vi "Write Card #.vi"(8 "error in (no error)":errorcluster, 10 "Card #":dbl, 11 "Universal Card in":refnum<class "Universal Card.lvclass">) -> (0 "error out":errorcluster, 3 "Universal Card out":refnum<class "Universal Card.lvclass">)   [LabVIEW 2012, in "Universal Power Meter.lvlib" / "Universal Card.lvclass"]
uses:
  Universal Card.lvclass
  Universal Card.lvclass/Universal Card.ctl
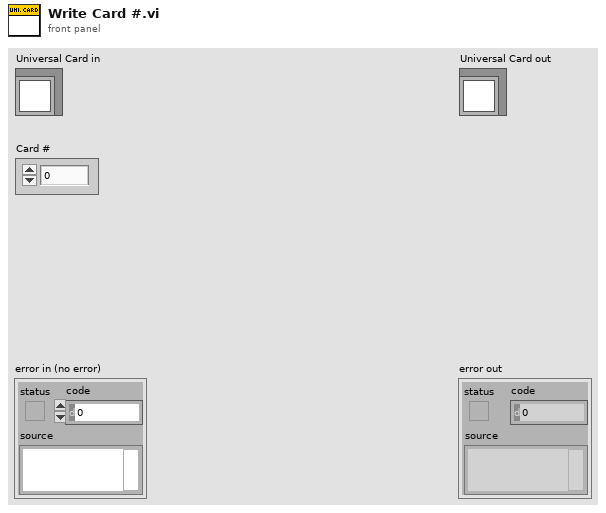
[diagram p1: front panel]
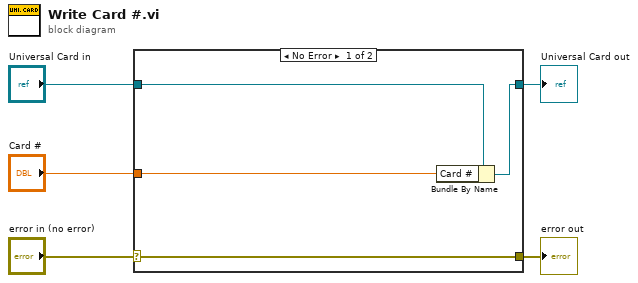
[diagram p0: block diagram]
diagram:
  n1 = case shown="No Error" "error in (no error)" {
    selector: "error in (no error)" -> [w9 w10]
    tunnel: [w9 w10] -> w4
    tunnel: [w7 w11] -> w2
    tunnel: "Universal Card in" -> [w8 w11]
    tunnel: "Card #" -> [w6 _]
    frame No Error {
      n2 = Bundle By Name(cluster=w8, "Card #"=w6) -> (w7:refnum<class "Universal Card.lvclass">)
    }
    frame Error {
    }
  }
  "error out" <- w4
  "Universal Card out" <- w2
